vi "Dvmg Start Configure Devices.vi"(8 "error in (no error)":errorcluster, 10 "perc":i32, 11 "hWnd":u32) -> (0 "error out":errorcluster, 2 "perc out":i32, 3 "hWnd out":u32)   [LabVIEW 2011, in "LVH-Adept.lvlib" / "DPCUTIL.lvlib"]
doc: "DPCAPI void DvmgStartConfigureDevices(HWND hWnd, ERC * perc);"
uses:
  DPCUTIL.lvlib
  <vilib>/LabVIEW Hacker/Adept/Private/Resources/dpcutil.dll
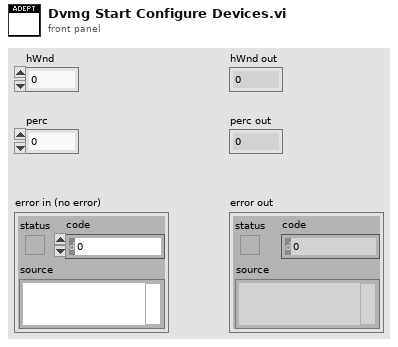
[diagram p1: front panel]
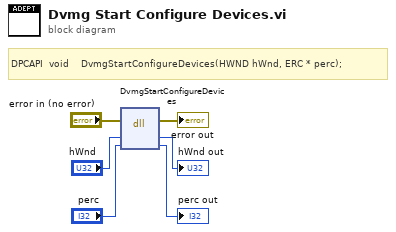
[diagram p0: block diagram]
diagram:
  # "DPCAPI  void    DvmgStartConfigureDevices(HWND hWnd, ERC * perc);"
  n1 = dll-call lib="C:/Program Files (x86)/National Instruments/LabVIEW 2011/vi.lib/LabVIEW Hacker/Adept/Private/Resources/dpcutil.*" fn="DvmgStartConfigureDevices"(error in="error in (no error)", "hWnd"="hWnd", "perc"="perc") -> (error out=→"error out":errorcluster, "hWnd"=→"hWnd out":u32, "perc"=→"perc out":i32)  [unwired: 3 in, 1 out]
